vi "Set Camera Origin.vi"(8 "error in (no error)":errorcluster, 10 "y":i32, 11 "x":i32) -> (0 "error out":errorcluster)   [LabVIEW 2018]
uses:
  LabSDL2/Source/Libraries/SDL2 Utility/Point (I32).ctl
  Re-use Libraries/Minimal Actor Framework/Messaging/Message/Message.lvclass/Message.ctl
  Globals.vi
  Re-use Libraries/Minimal Actor Framework/Messaging/Message/Message.lvclass
  Main Controller Actor API.lvclass
  LabSDL2/Source/Libraries/SDL2 Utility/SDL2 Utility.lvlib
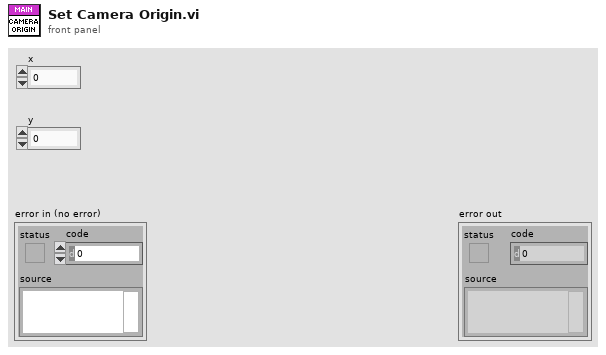
[diagram p1: front panel]
types:
  T1 = typedef "SDL2 Utility.lvlib/Point (I32).ctl" = cluster{"x":i32, "y":i32}
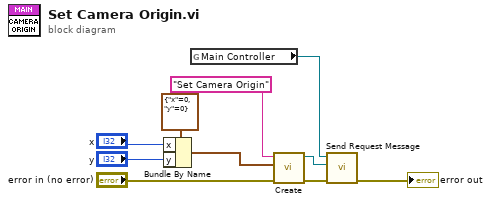
[diagram p0: block diagram]
diagram:
  n1 = Bundle By Name(cluster=T1 {"x"=0, "y"=0} ("Point"), "x"="x", "y"="y") -> (w3:T1)
  n2 = global read "Globals.vi" "Main Controller"() -> (w7:refnum<class "Main Controller Actor API.lvclass">)
  n3 = call "Create.vi"("error in (no error)"="error in (no error)", "Data"=w3, "Name"="Set Camera Origin" ("Parameter")) -> ("error out"=w8:errorcluster, "Message out"=w9:refnum<class "Message.lvclass">)  [unwired: 7 in]
  n4 = call-dynamic "Send Request Message.vi"("error in (no error)"=w8, "Message"=w9, "Actor API in"=w7) -> ("error out"=→"error out":errorcluster)  [unwired: 8 in]
